vi "Events to table.vi"(8 "error in (no error)":errorcluster, 11 "references in":T1) -> (0 "error out":errorcluster, 2 "table":string[][](array[string]), 3 "references out":T1)   [LabVIEW 2013, in "tag select module editor node.lvclass"]
uses:
  tag select module editor node.lvclass
  references.ctl
  <vilib>/NI/Configuration Framework/Node/StopEvent.ctl
  <vilib>/NI/Configuration Framework/Node/RefreshUIEvent.ctl
  <vilib>/NI/Configuration Framework/Node/CacheState.ctl
  <vilib>/NI/Configuration Framework/Node/NodeChangeEvent.ctl
  <vilib>/NI/Configuration Framework/Node/NodeRef.ctl
  <vilib>/NI/Configuration Framework/Node/NISE_CEF_Node.lvclass
  <vilib>/NI/Tag Bus Data Framework/control module/editor node/channel action event.ctl
  <vilib>/NI/Tag Bus Data Framework/control module/editor node/dialog output action.ctl
  <vilib>/NI/Tag Bus Module Framework/channel/TBM channel.lvclass
  <vilib>/NI/Tag Bus/tag/tag descriptor.lvclass
  <vilib>/NI/AMC/Message Queue.ctl
  <vilib>/NI/AMC/Message.ctl
  <vilib>/NI/Tools/Keyed Array/KeyedArray.ctl
  <vilib>/NI/Tag Bus Data Framework/Configuration Editor/Classes/Engine Parent/Engine Parent Editor Node.lvclass
  module/configuration/tag select module configuration.lvclass
  <vilib>/NI/Tag Bus Data Framework/Configuration Editor/Classes/Engine Parent/read engine configuration.vi
  <vilib>/NI/Tag Bus Data Framework/Configuration Editor/Classes/Module editor node/Read Module Configuration.vi
  <vilib>/NI/Module Execution Interface/Engine Configuration/engine configuration.lvclass
  <vilib>/NI/Tag Bus Module Framework/module configuration/TBM module configuration.lvclass
  <vilib>/NI/Tag Bus Data Framework/control module/editor node/control module editor.lvclass
  <vilib>/NI/Tools/Keyed Array/Tools_KeyedArray.lvlib
  <vilib>/NI/AMC/AMC.lvlib
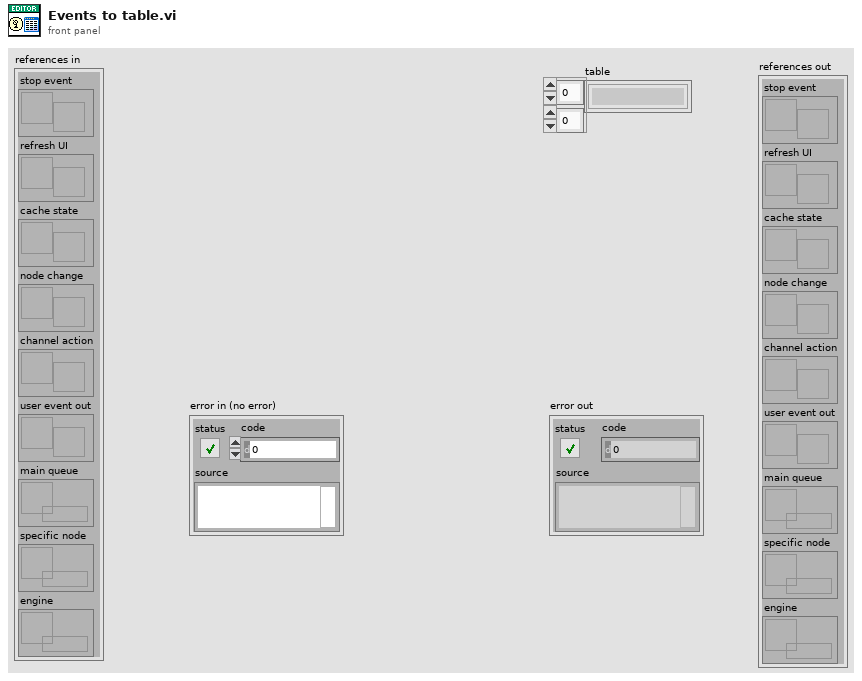
[diagram p1: front panel]
types:
  T1 = typedef "tag select module editor node.lvclass/references.ctl" = cluster{"stop event":T2, "refresh UI":T3, "cache state":T4, "node change":T5, "channel action":refnum<user-event>, "user event out":refnum<user-event>, "main queue":T6, "specific node":refnum<data-value>, "engine":refnum<data-value>}
  T2 = typedef "NISE_CEF_Node.lvclass/StopEvent.ctl" = refnum<user-event>
  T3 = typedef "NISE_CEF_Node.lvclass/RefreshUIEvent.ctl" = refnum<user-event>
  T4 = typedef "NISE_CEF_Node.lvclass/CacheState.ctl" = refnum<user-event>
  T5 = typedef "NISE_CEF_Node.lvclass/NodeChangeEvent.ctl" = refnum<user-event>
  T6 = typedef "AMC.lvlib/Message Queue.ctl" = refnum<queue>
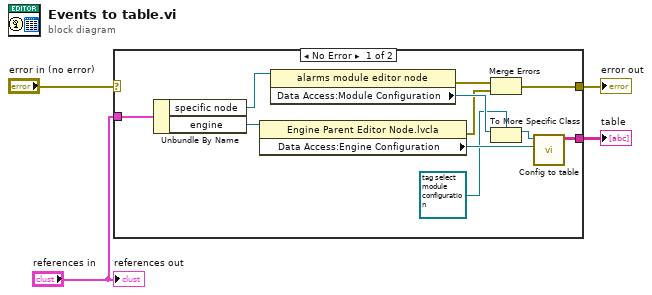
[diagram p0: block diagram]
diagram:
  n1 = case shown="No Error" "error in (no error)" {
    selector: "error in (no error)" -> [_ w16]
    tunnel: [w15 _] -> w4
    tunnel: "references in" -> [w8 _]
    tunnel: [w5 w16] -> w1
    frame No Error {
      n2 = Unbundle By Name(w8) -> ("specific node"=w13:refnum<data-value>, "engine"=w14:refnum<data-value>)
      n3 = property class="Engine Parent Editor Node.lvcla"(reference=w14) -> (error out=w7:errorcluster, "Data Access:Engine Configuration"=w12:refnum<class "engine configuration.lvclass">)  [unwired: 1 in, 1 out]
      n4 = property class="alarms module editor node"(reference=w13) -> (error out=w6:errorcluster, "Data Access:Module Configuration"=w11:refnum<class "TBM module configuration.lvclass">)  [unwired: 1 in, 1 out]
      n5 = Merge Errors(w6, w7) -> (w5:errorcluster)
      n6 = To More Specific Class(target class=refnum<class "tag select module configuration.lvclass"> refnum ("tag select module configuration in"), reference=w11) -> (specific class reference=w9:refnum<class "tag select module configuration.lvclass">)  [unwired: 1 in, 1 out]
      n7 = call "Config to table.vi"("engine configuration"=w12, "tag select module configuration in"=w9) -> ("Array"=w15:string[][])  [unwired: 9 in]
    }
    frame Error {
    }
  }
  "table" <- w4
  "error out" <- w1
  "references out" <- "references in"
